vi "Refresh.vi"(8 "error in (no error)":errorcluster, 11 "Configuration":T1) -> (0 "error out":errorcluster)   [LabVIEW 2013, in "LVTM.lvlib"]
uses:
  LVTM.lvlib
  Controls_LVTM/LVTM_Config_Info.ctl
  Controls_LVTM/View.ctl
  Controls_LVTM/SharedDataDVR.ctl
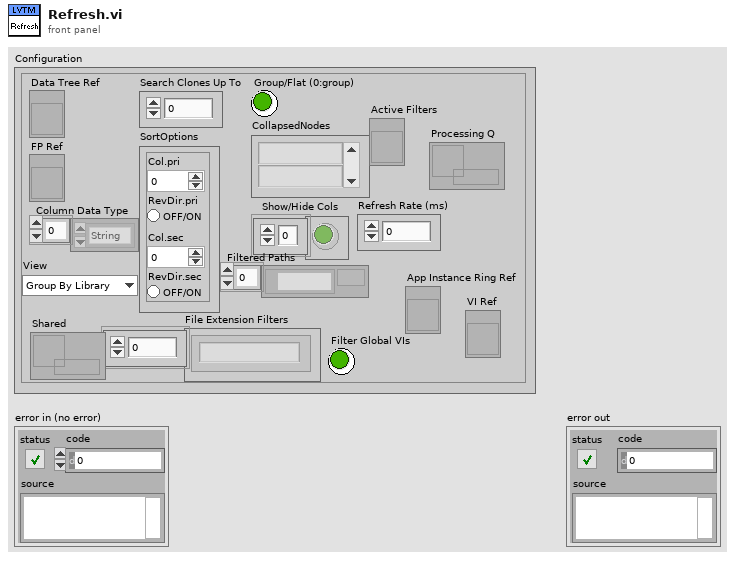
[diagram p1: front panel]
types:
  T1 = typedef "LVTM.lvlib/LVTM_Config_Info.ctl" = cluster{"Data Tree Ref":refnum<vi>, "FP Ref":refnum<vi>, "Column Data Type":enum16{"String", "Numeric"}[], "Search Clones Up To":i32, "SortOptions":cluster{"Col.pri":i32, "RevDir.pri":bool, "Col.sec":i32, "RevDir.sec":bool}, "Group/Flat (0:group)":bool, "CollapsedNodes":string[], "Show/Hide Cols":bool[], "Filtered Paths":path[], "View":T2, "File Extension Filters":string[], "Filter Global VIs":bool, "Shared":refnum<data-value>, "Active Filters":refnum<vi>, "Refresh Rate (ms)":i32, "App Instance Ring Ref":refnum<vi>, "Processing Q":refnum<queue>, "VI Ref":refnum<vi>}
  T2 = typedef "LVTM.lvlib/View.ctl" = enum16{"Group By Library", "Group By Folder", "Flat List"}
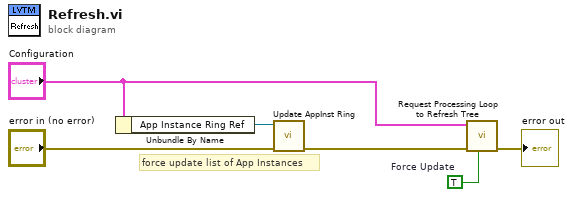
[diagram p0: block diagram]
diagram:
  w4 = TRUE  # Force Update
  # "force update list of App Instances"
  n1 = Unbundle By Name("Configuration") -> ("App Instance Ring Ref"=w6:refnum<vi>)
  n2 = call "Update AppInst Ring.vi"("error in"="error in (no error)", "Ring in"=w6) -> ("error out"=w2:errorcluster)  [unwired: 7 in, 2 out]
  n3 = call "Request Processing Loop to Refresh Tree.vi"("Force Update"=w4, "error in (no error)"=w2, "ConfigInfo in"="Configuration") -> ("error out"=→"error out":errorcluster)  [unwired: 8 in]
